vi "Extract Designated Orders.vi"(6 "window info":T1={"window type"=10, "window length"=2048} {"window type" items=["None"=0, "Hanning"=1, "Hamming"=2, "Blackman-Harris"=3, "Exact Blackman"=4, "Blackman"=5, "Flat Top"=6, "4 Term B-Harris"=7, "7 Term B-Harris"=8, "Low Sidelobe"=9, "Gaussian"=62]; "window length" min=0}, 7 "bandwidth":T2={"bandwidth value"=0.5, "bandwidth unit"=enum."Order"} {"bandwidth value" min=0.0 format="%.2f"}, 8 "error in (no error)":errorcluster, 9 "orders (1.0)":dbl[](array[numeric])=[1.0] format="%.2f", 10 "speed profile":T3 {"speed [RPM]" format="%.2f"; "time [s]" format="%.2f"}, 11 "scaled signal [EU]":waveform(dbl)={"t0"=timestamp(0 s since 1904-01-01), "dt"=0.0, "Y"=[]}) -> (0 "error out":errorcluster, 1 "unit label":string, 3 "order waveforms [EU]":waveform(dbl)[](array[waveform]), 4 "actual window":T1={"window type"=10, "window length"=2048} {"window type" items=["None"=0, "Hanning"=1, "Hamming"=2, "Blackman-Harris"=3, "Exact Blackman"=4, "Blackman"=5, "Flat Top"=6, "4 Term B-Harris"=7, "7 Term B-Harris"=8, "Low Sidelobe"=9, "Gaussian"=62]; "window length" min=0})   [LabVIEW 2017]
doc: "Extracts orders from <B>scaled signal [EU]</B>."
uses:
  <vilib>/addons/Sound and Vibration/Order Analysis/Tach Process/SubVIs/speed profile.ctl
  <vilib>/addons/Sound and Vibration/Order Analysis/Ref Gabor Order Tracking/Mask Bandwidth.ctl
  <vilib>/addons/Sound and Vibration/Order Analysis/Ref Gabor Order Tracking/window information.ctl
  <vilib>/addons/_NISVFA/_Shared subVIs/Common/svc_Engineering Units to Unit Label.vi
  <vilib>/addons/_NISVFA/_Shared subVIs/Common/svc_Unit Label to Engineering Units.vi
  <vilib>/addons/Sound and Vibration/Order Analysis/Gabor Order Tracking/SoundVib_Gabor.lvlib
  <vilib>/addons/Sound and Vibration/Order Analysis/Tach Process/SoundVib_TachProcess.lvlib
panel:
  # "Extract Designated Orders"
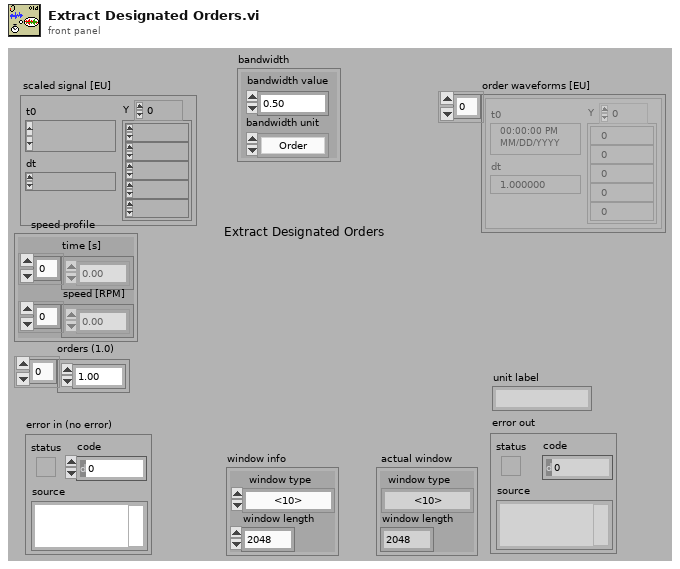
[diagram p1: front panel]
types:
  T1 = typedef "SoundVib_Gabor.lvlib/window information.ctl" = cluster{"window type":u32, "window length":i32}
  T2 = typedef "SoundVib_Gabor.lvlib/Mask Bandwidth.ctl" = cluster{"bandwidth value":dbl, "bandwidth unit":enum16{"Order", "Hz"}}
  T3 = typedef "SoundVib_TachProcess.lvlib/speed profile.ctl" = cluster{"time [s]":dbl[], "speed [RPM]":dbl[]}
  T4 = typedef "svc_Channel Info.ctl" = cluster{"sensor sensitivity":dbl, "engineering units":T5, "dB reference":dbl, "custom label":string, "weighting filter":T6, "pregain":dbl}
  T5 = typedef "svc_Engineering Units Text Ring.ctl" = u16
  T6 = typedef "svc_Weighting Filter Text Ring.ctl" = u16
  T7 = typedef "SoundVib_Gabor.lvlib/GT RefNum.ctl" = refnum<k1>
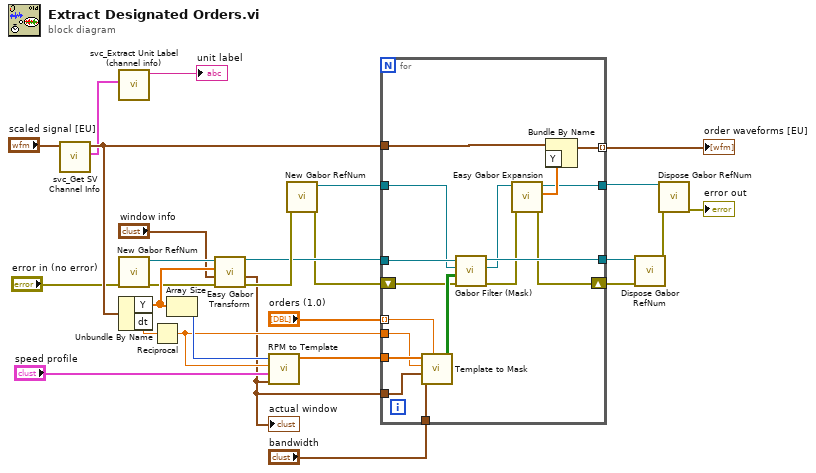
[diagram p0: block diagram]
diagram:
  n1 = call <vilib>:"svc_Get SV Channel Info.vi"("scaled signal [EU]"="scaled signal [EU]") -> ("channel info"=w12:T4, "dup scaled signal [EU]"=w13:waveform(dbl))  [unwired: 5 in, 4 out]
  n2 = call <vilib>:"svc_Extract Unit Label (channel info).vi"("channel info"=w12) -> ("unit label"=→"unit label":string)  [unwired: 8 in, 2 out]
  n3 = call <vilib>:"New Gabor RefNum.vi"("error in (no error)"="error in (no error)") -> ("error out"=w6:errorcluster, "RefNum"=w9:T7)  [unwired: 8 in]
  n4 = Unbundle By Name(w13) -> ("Y"=w8:dbl[], "dt"=w17:dbl)
  n5 = Reciprocal(x=w17) -> (1/x=w18:dbl)
  n6 = Array Size(array=w8) -> (size(s)=w24:i32)
  n7 = call <vilib>:"Easy Gabor Transform.vi"("error in (no error)"=w6, "window info"="window info", "x[n]"=w8, "RefNum in"=w9) -> ("error out"=w5:errorcluster, "actual window"=w4:T1, "RefNum out"=w3:T7)  [unwired: 3 in, 2 out]
  "actual window" <- w4
  n8 = call <vilib>:"RPM to Template.vi"("window info"=w4, "speed profile"="speed profile", "sampling frequency [Hz]"=w18, "signal length"=w24) -> ("Gabor template"=w26:dbl[])  [unwired: 6 in, 1 out]
  n9 = call <vilib>:"New Gabor RefNum.vi"("error in (no error)"=w5) -> ("error out"=w2:errorcluster, "RefNum"=w27:T7)  [unwired: 8 in]
  n10 = for {
    tunnel: w3 -> [w44]
    tunnel: w27 -> [w43]
    tunnel: [w42] -> w11
    tunnel: [w30] -> w10
    tunnel: w26 -> [w41]
    tunnel: "orders (1.0)" -> [w39] mode=indexing
    shift-right: [w28] -> w23
    shift-left: w2 -> [w38]
    tunnel: [w29] -> w16 mode=indexing
    tunnel: "bandwidth" -> [w34]
    tunnel: w18 -> [w35]
    tunnel: w13 -> [w33]
    tunnel: w4 -> [w31]
    n11 = call <vilib>:"Template to Mask.vi"("order (1.0)"=w39, "bandwidth"=w34, "window info"=w31, "sampling frequency [S/s]"=w35, "Gabor template"=w41) -> ("mask array"=w40:bool[][])  [unwired: 6 in]
    n12 = call <vilib>:"Gabor Filter (Mask).vi"("error in (no error)"=w38, "mask array"=w40, "dest RefNum in"=w43, "src RefNum in"=w44) -> ("error out"=w36:errorcluster, "dest RefNum out"=w37:T7, "RefNum out"=w42:T7)  [unwired: 5 in]
    n13 = call <vilib>:"Easy Gabor Expansion.vi"("error in (no error)"=w36, "RefNum in"=w37) -> ("error out"=w28:errorcluster, "time waveform"=w32:dbl[], "RefNum out"=w30:T7)  [unwired: 7 in]
    n14 = Bundle By Name(cluster=w33, "Y"=w32) -> (w29:waveform(dbl))
  }
  "order waveforms [EU]" <- w16
  n15 = call <vilib>:"Dispose Gabor RefNum.vi"("error in (no error)"=w23, "RefNum in"=w11) -> ("error out"=w22:errorcluster)  [unwired: 6 in]
  n16 = call <vilib>:"Dispose Gabor RefNum.vi"("error in (no error)"=w22, "RefNum in"=w10) -> ("error out"=→"error out":errorcluster)  [unwired: 6 in]
